vi "Configuration Changed.vi"(8 "error in (no error)":errorcluster, 10 "Canceled? (F)":bool, 11 "Cfg Grandmaster in":refnum<class "Cfg Grandmaster.lvclass">) -> (0 "error out":errorcluster, 3 "Cfg Grandmaster out":refnum<class "Cfg Grandmaster.lvclass">)   [LabVIEW 2012, in "Configuration Grandmaster.lvlib" / "Cfg Grandmaster.lvclass"]
uses:
  Cfg Grandmaster.lvclass
  Cfg Grandmaster.lvclass/Cfg Grandmaster.ctl
  Class FP Ctrls/FP Controls.lvclass
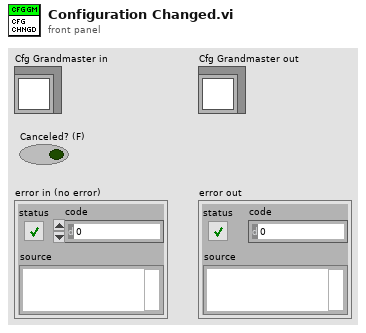
[diagram p1: front panel]
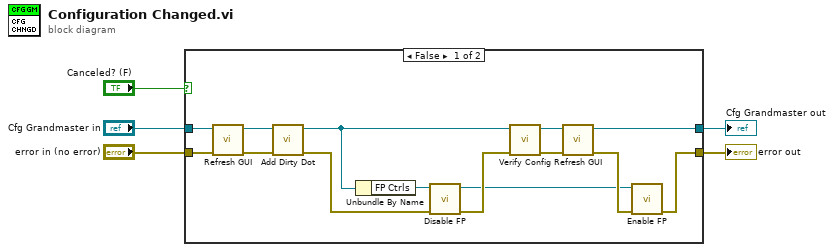
[diagram p0: block diagram]
diagram:
  n1 = case shown="False" "Canceled? (F)" {
    tunnel: [w9 w21] -> w4
    tunnel: "error in (no error)" -> [w19 w21]
    tunnel: "Cfg Grandmaster in" -> [w16 w20]
    tunnel: [w13 w20] -> w5
    frame False {
      n2 = call "Refresh GUI.vi"("error in (no error)"=w19, "Cfg Grandmaster in"=w16) -> ("error out"=w18:errorcluster, "Cfg Grandmaster out"=w15:refnum<class "Cfg Grandmaster.lvclass">)  [unwired: 8 in]
      n3 = call "Add Dirty Dot.vi"("error in (no error)"=w18, "Cfg Grandmaster in"=w15) -> ("error out"=w12:errorcluster, "Cfg Grandmaster out"=w6:refnum<class "Cfg Grandmaster.lvclass">)  [unwired: 7 in, 1 out]
      n4 = Unbundle By Name(w6) -> ("FP Ctrls"=w8:refnum<class "FP Controls.lvclass">)
      n5 = call "Disable FP.vi"("error in (no error)"=w12, "FP Controls in"=w8) -> ("error out"=w11:errorcluster, "FP Controls out"=w7:refnum<class "FP Controls.lvclass">)  [unwired: 8 in]
      n6 = call "Verify Config.vi"("error in (no error)"=w11, "Cfg Grandmaster in"=w6) -> ("error out"=w17:errorcluster, "Cfg Grandmaster out"=w14:refnum<class "Cfg Grandmaster.lvclass">)  [unwired: 8 in]
      n7 = call "Refresh GUI.vi"("error in (no error)"=w17, "Cfg Grandmaster in"=w14) -> ("error out"=w10:errorcluster, "Cfg Grandmaster out"=w13:refnum<class "Cfg Grandmaster.lvclass">)  [unwired: 8 in]
      n8 = call "Enable FP.vi"("error in (no error)"=w10, "FP Controls in"=w7) -> ("error out"=w9:errorcluster)  [unwired: 8 in, 1 out]
    }
    frame True {
    }
  }
  "Cfg Grandmaster out" <- w5
  "error out" <- w4
